vi "PumpDispense.vi"(8 "Error In":errorcluster, 9 "Flowrate(ul/min)":dbl, 10 "Pump Address":string, 11 "Pump COMM Port":refnum<visa-resource-name>) -> (0 "Error Out":errorcluster, 3 "Pump COMM Port Out":refnum<visa-resource-name>)   [LabVIEW 2015]
panel:
  # "Dispense Micro Lynx Milligat Pumps"
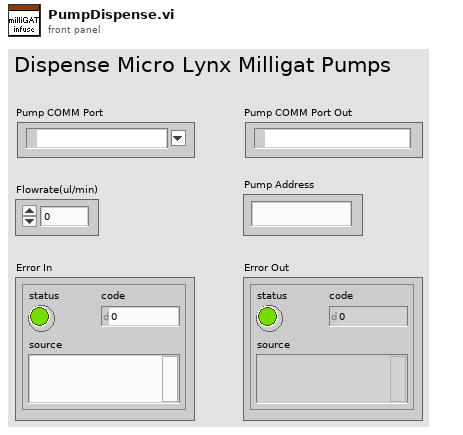
[diagram p1: front panel]
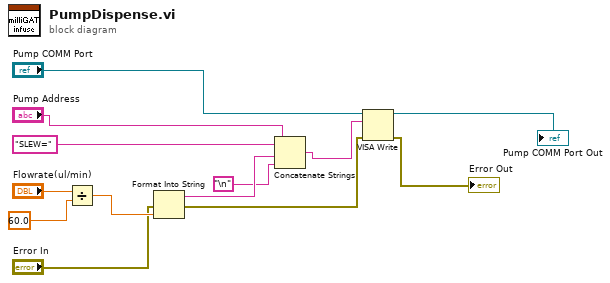
[diagram p0: block diagram]
diagram:
  n1 = Divide(x="Flowrate(ul/min)", y=60.0) -> (x/y=w10:dbl)
  n2 = Format Into String(error in="Error In", w10) -> (resulting string=w3:string, error out=w8:errorcluster)  [unwired: 2 in]
  n3 = Concatenate Strings("Pump Address", "SLEW=", w3, "\n") -> (w6:string)
  n4 = VISA Write(VISA resource name="Pump COMM Port", write buffer=w6, error in (no error)=w8) -> (VISA resource name out=→"Pump COMM Port Out":refnum<visa-resource-name>, error out=→"Error Out":errorcluster)  [unwired: 1 out]
